vi "bottom player court segment(SubVI).vi"(10 "Bottom player position":cluster{"Numeric":dbl, "Numeric":dbl}[](array[cluster]), 11 "previous segment":i32) -> (2 "Bottom player segment position":string)   [LabVIEW 2013]
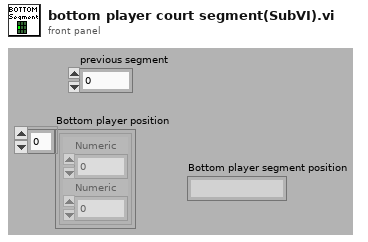
[diagram p1: front panel]
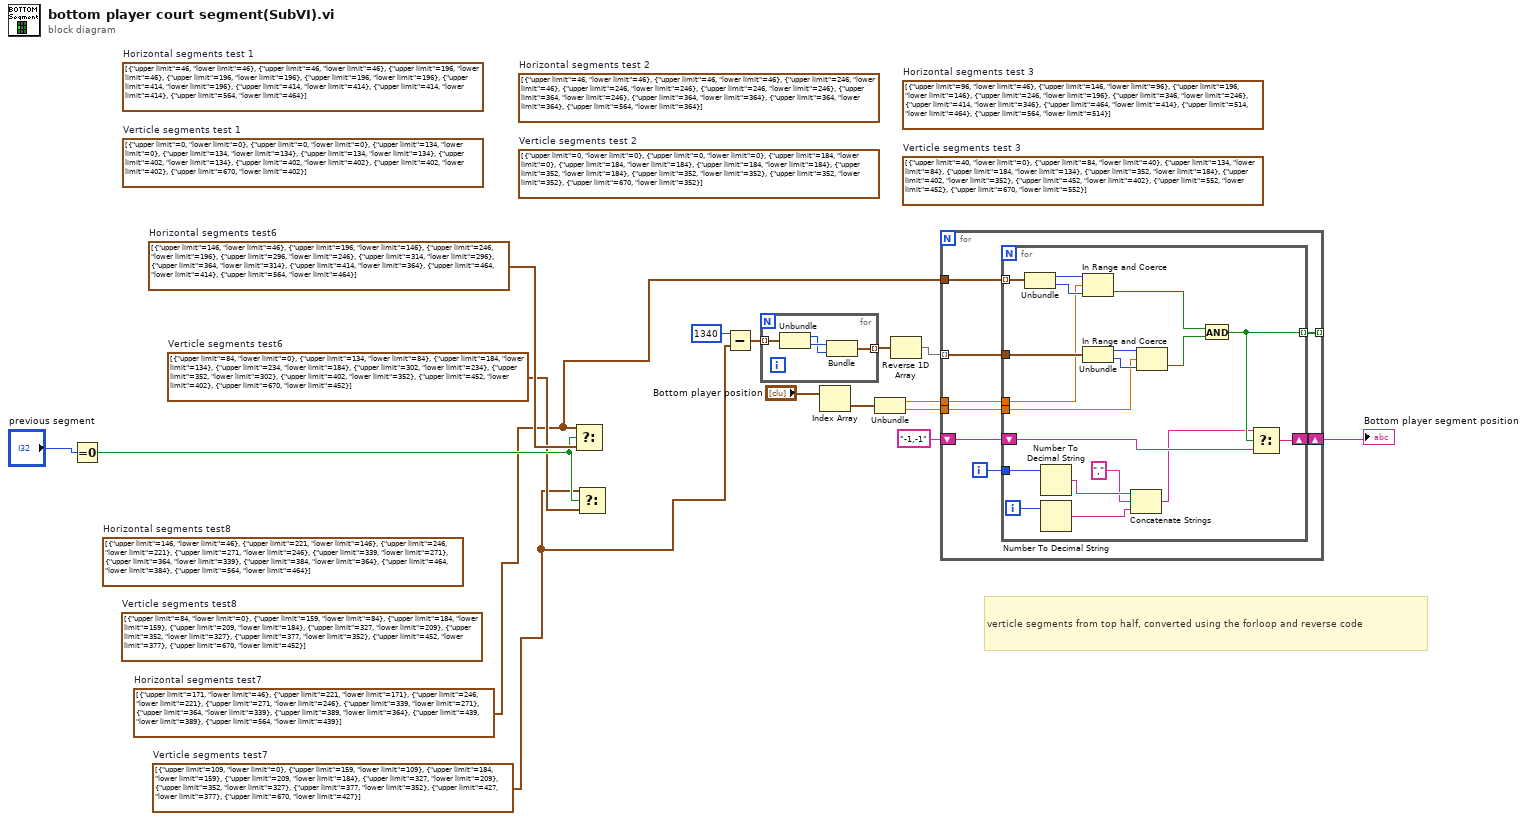
[diagram p0: block diagram]
diagram:
  (unwired) cluster{"upper limit":i32, "lower limit":i32}[] [{"upper limit"=146, "lower limit"=46}, {"upper limit"=221, "lower limit"=146}, {"upper limit"=246, "lower limit"=221}, {"upper limit"=271, "lower limit"=246}, {"upper limit"=339, "lower limit"=271}, {"upper limit"=364, "lower limit"=339}, {"upper limit"=384, "lower limit"=364}, {"upper limit"=464, "lower limit"=384}, {"upper limit"=564, "lower limit"=464}]  # Horizontal segments test8
  (unwired) cluster{"upper limit":i32, "lower limit":i32}[] [{"upper limit"=84, "lower limit"=0}, {"upper limit"=159, "lower limit"=84}, {"upper limit"=184, "lower limit"=159}, {"upper limit"=209, "lower limit"=184}, {"upper limit"=327, "lower limit"=209}, {"upper limit"=352, "lower limit"=327}, {"upper limit"=377, "lower limit"=352}, {"upper limit"=452, "lower limit"=377}, {"upper limit"=670, "lower limit"=452}]  # Verticle segments test8
  w1 = cluster{"upper limit":i32, "lower limit":i32}[] [{"upper limit"=171, "lower limit"=46}, {"upper limit"=221, "lower limit"=171}, {"upper limit"=246, "lower limit"=221}, {"upper limit"=271, "lower limit"=246}, {"upper limit"=339, "lower limit"=271}, {"upper limit"=364, "lower limit"=339}, {"upper limit"=389, "lower limit"=364}, {"upper limit"=439, "lower limit"=389}, {"upper limit"=564, "lower limit"=439}]  # Horizontal segments test7
  w2 = cluster{"upper limit":i32, "lower limit":i32}[] [{"upper limit"=109, "lower limit"=0}, {"upper limit"=159, "lower limit"=109}, {"upper limit"=184, "lower limit"=159}, {"upper limit"=209, "lower limit"=184}, {"upper limit"=327, "lower limit"=209}, {"upper limit"=352, "lower limit"=327}, {"upper limit"=377, "lower limit"=352}, {"upper limit"=427, "lower limit"=377}, {"upper limit"=670, "lower limit"=427}]  # Verticle segments test7
  (unwired) cluster{"upper limit":i32, "lower limit":i32}[] [{"upper limit"=40, "lower limit"=0}, {"upper limit"=84, "lower limit"=40}, {"upper limit"=134, "lower limit"=84}, {"upper limit"=184, "lower limit"=134}, {"upper limit"=352, "lower limit"=184}, {"upper limit"=402, "lower limit"=352}, {"upper limit"=452, "lower limit"=402}, {"upper limit"=552, "lower limit"=452}, {"upper limit"=670, "lower limit"=552}]  # Verticle segments test 3
  (unwired) cluster{"upper limit":i32, "lower limit":i32}[] [{"upper limit"=96, "lower limit"=46}, {"upper limit"=146, "lower limit"=96}, {"upper limit"=196, "lower limit"=146}, {"upper limit"=246, "lower limit"=196}, {"upper limit"=346, "lower limit"=246}, {"upper limit"=414, "lower limit"=346}, {"upper limit"=464, "lower limit"=414}, {"upper limit"=514, "lower limit"=464}, {"upper limit"=564, "lower limit"=514}]  # Horizontal segments test 3
  (unwired) cluster{"upper limit":i32, "lower limit":i32}[] [{"upper limit"=0, "lower limit"=0}, {"upper limit"=0, "lower limit"=0}, {"upper limit"=184, "lower limit"=0}, {"upper limit"=184, "lower limit"=184}, {"upper limit"=184, "lower limit"=184}, {"upper limit"=352, "lower limit"=184}, {"upper limit"=352, "lower limit"=352}, {"upper limit"=352, "lower limit"=352}, {"upper limit"=670, "lower limit"=352}]  # Verticle segments test 2
  (unwired) cluster{"upper limit":i32, "lower limit":i32}[] [{"upper limit"=46, "lower limit"=46}, {"upper limit"=46, "lower limit"=46}, {"upper limit"=246, "lower limit"=46}, {"upper limit"=246, "lower limit"=246}, {"upper limit"=246, "lower limit"=246}, {"upper limit"=364, "lower limit"=246}, {"upper limit"=364, "lower limit"=364}, {"upper limit"=364, "lower limit"=364}, {"upper limit"=564, "lower limit"=364}]  # Horizontal segments test 2
  (unwired) cluster{"upper limit":i32, "lower limit":i32}[] [{"upper limit"=0, "lower limit"=0}, {"upper limit"=0, "lower limit"=0}, {"upper limit"=134, "lower limit"=0}, {"upper limit"=134, "lower limit"=134}, {"upper limit"=134, "lower limit"=134}, {"upper limit"=402, "lower limit"=134}, {"upper limit"=402, "lower limit"=402}, {"upper limit"=402, "lower limit"=402}, {"upper limit"=670, "lower limit"=402}]  # Verticle segments test 1
  (unwired) cluster{"upper limit":i32, "lower limit":i32}[] [{"upper limit"=46, "lower limit"=46}, {"upper limit"=46, "lower limit"=46}, {"upper limit"=196, "lower limit"=46}, {"upper limit"=196, "lower limit"=196}, {"upper limit"=196, "lower limit"=196}, {"upper limit"=414, "lower limit"=196}, {"upper limit"=414, "lower limit"=414}, {"upper limit"=414, "lower limit"=414}, {"upper limit"=564, "lower limit"=464}]  # Horizontal segments test 1
  w5 = cluster{"upper limit":i32, "lower limit":i32}[] [{"upper limit"=146, "lower limit"=46}, {"upper limit"=196, "lower limit"=146}, {"upper limit"=246, "lower limit"=196}, {"upper limit"=296, "lower limit"=246}, {"upper limit"=314, "lower limit"=296}, {"upper limit"=364, "lower limit"=314}, {"upper limit"=414, "lower limit"=364}, {"upper limit"=464, "lower limit"=414}, {"upper limit"=564, "lower limit"=464}]  # Horizontal segments test6
  w3 = cluster{"upper limit":i32, "lower limit":i32}[] [{"upper limit"=84, "lower limit"=0}, {"upper limit"=134, "lower limit"=84}, {"upper limit"=184, "lower limit"=134}, {"upper limit"=234, "lower limit"=184}, {"upper limit"=302, "lower limit"=234}, {"upper limit"=352, "lower limit"=302}, {"upper limit"=402, "lower limit"=352}, {"upper limit"=452, "lower limit"=402}, {"upper limit"=670, "lower limit"=452}]  # Verticle segments test6
  # "verticle segments from top half, converted using the forloop and reverse code"
  n1 = Equal To 0?(x="previous segment") -> (x = 0?=w4:bool)
  n2 = Select(t=w1, s=w4, f=w5) -> ()  [unwired: 1 out]
  n3 = Select(t=w2, s=w4, f=w3) -> ()  [unwired: 1 out]
  n4 = Subtract(x=1340 ("upper limit"), y=w2) -> (x-y=w10:cluster{"upper limit":i32, "lower limit":i32}[])
  n5 = for {
    tunnel: w10 -> [w17] mode=indexing
    tunnel: [w18] -> w9 mode=indexing
    n6 = Unbundle(w17) -> ("upper limit"=w19:i32, "lower limit"=w20:i32)
    n7 = Bundle("lower limit"=w20, "upper limit"=w19) -> (w18:cluster{"lower limit":i32, "upper limit":i32})  [unwired: 1 in]
  }
  n8 = Index Array(array="Bottom player position") -> (element=w15:cluster{"Numeric":dbl, "Numeric":dbl})  [unwired: 1 in]
  n9 = Unbundle(w15) -> ("Numeric"=w13:dbl, "Numeric"=w14:dbl)
  n10 = Reverse 1D Array(array=w9) -> (reversed array=w8:cluster{"lower limit":i32, "upper limit":i32}[])
  n11 = for {
    tunnel: w8 -> [w27] mode=indexing
    tunnel: w1 -> [w28]
    tunnel: w14 -> [w26]
    tunnel: w13 -> [w25]
    tunnel: [w24] -> _ mode=indexing
    shift-right: [w22] -> w11
    shift-left: "-1,-1" ("decimal integer string") -> [w21]
    i -> [w23]
    n12 = for {
      tunnel: w28 -> [w47] mode=indexing
      tunnel: w27 -> [w46]
      tunnel: w26 -> [w41]
      tunnel: w25 -> [w40]
      tunnel: [w37] -> w24 mode=indexing
      tunnel: w23 -> [w34]
      shift-right: [w36] -> w22
      shift-left: w21 -> [w35]
      i -> [w33]
      n13 = Unbundle(w47) -> ("upper limit"=w45:i32, "lower limit"=w44:i32)
      n14 = Number To Decimal String(number=w34) -> (decimal integer string=w32:string)  [unwired: 1 in]
      n15 = Number To Decimal String(number=w33) -> (decimal integer string=w30:string)  [unwired: 1 in]
      n16 = In Range and Coerce(upper limit=w45, x=w40, lower limit=w44) -> (In Range?=w39:bool)  [unwired: 1 out]
      n17 = Unbundle(w46) -> ("lower limit"=w43:i32, "upper limit"=w42:i32)
      n18 = Concatenate Strings(w32, "," ("string"), w30) -> (w31:string)
      n19 = In Range and Coerce(upper limit=w43, x=w41, lower limit=w42) -> (In Range?=w38:bool)  [unwired: 1 out]
      n20 = And(x=w39, y=w38) -> (x .and. y?=w37:bool)
      n21 = Select(t=w31, s=w37, f=w35) -> (s? t:f=w36:string)
    }
  }
  "Bottom player segment position" <- w11
